vi "Function code mismatch error.vi"(8 "error in (no error)":errorcluster) -> (0 "error out":errorcluster)   [LabVIEW 2018, in "SubVIs.lvlib" / "Master Function Definition.lvlib"]
uses:
  Master Function Definition.lvlib
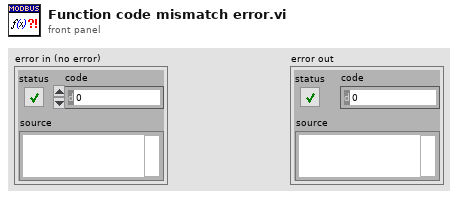
[diagram p1: front panel]
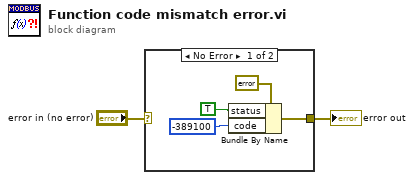
[diagram p0: block diagram]
diagram:
  n1 = case shown="No Error" "error in (no error)" {
    selector: "error in (no error)" -> [_ w7]
    tunnel: [w3 w7] -> w1
    frame No Error {
      n2 = Bundle By Name(cluster=errorcluster {"status"=FALSE, "code"=0, "source"=""} ("error constant"), "status"=TRUE, "code"=-389100) -> (w3:errorcluster)
    }
    frame Error {
    }
  }
  "error out" <- w1
